vi "RelaySafetyTest.vi"(0 "Relay Task":refnum<k21>, 5 "task error in":errorcluster, 9 "NI VISA":refnum<visa-resource-name>, 11 "NHR error in":errorcluster caption="error in (no error)") -> (6 "error out":errorcluster, 8 "Safe to connect":bool, 10 "NHR Visa out":refnum<visa-resource-name>, 15 "NHR error out":errorcluster)   [LabVIEW 2020]
uses:
  <vilib>/DAQmx/write.llb/DAQmx Write (Digital 1D Bool NChan 1Samp 1Line).vi
  <vilib>/DAQmx/miscellaneous.llb/DAQmx Fill In Error Info.vi
  <instrlib>/NH Research Regenerative Test Series/Public/Data/Read (Ave Voltage).vi
  <instrlib>/NH Research Regenerative Test Series/NH Research Regenerative Test Series.lvlib
panel:
  out "Ave Voltage (V) 3":dbl
  out "Ave Voltage (V) 2":dbl
  out "Ave Voltage (V) 1":dbl
  in  "Logical Instrument Number":u32=1
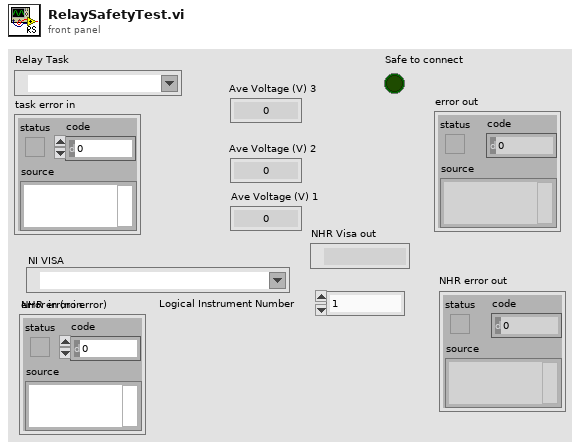
[diagram p1: front panel]
types:
  T1 = cluster{"Min Voltage (V)":dbl, "Min Voltage Time (s)":dbl, "Max Voltage (V)":dbl, "Max Voltage Time (s)":dbl, "Max Sink Current (A)":dbl, "Max Sink Current Time (s)":dbl, "Max Source Current (A)":dbl, "Max Source Current Time (s)":dbl, "Max Sink Power (W)":dbl, "Max Sink Power Time (s)":dbl, "Max Source Power (W)":dbl, "Max Source Power Time (s)":dbl}
  T2 = cluster{bool, bool, bool, bool, bool, bool, bool}
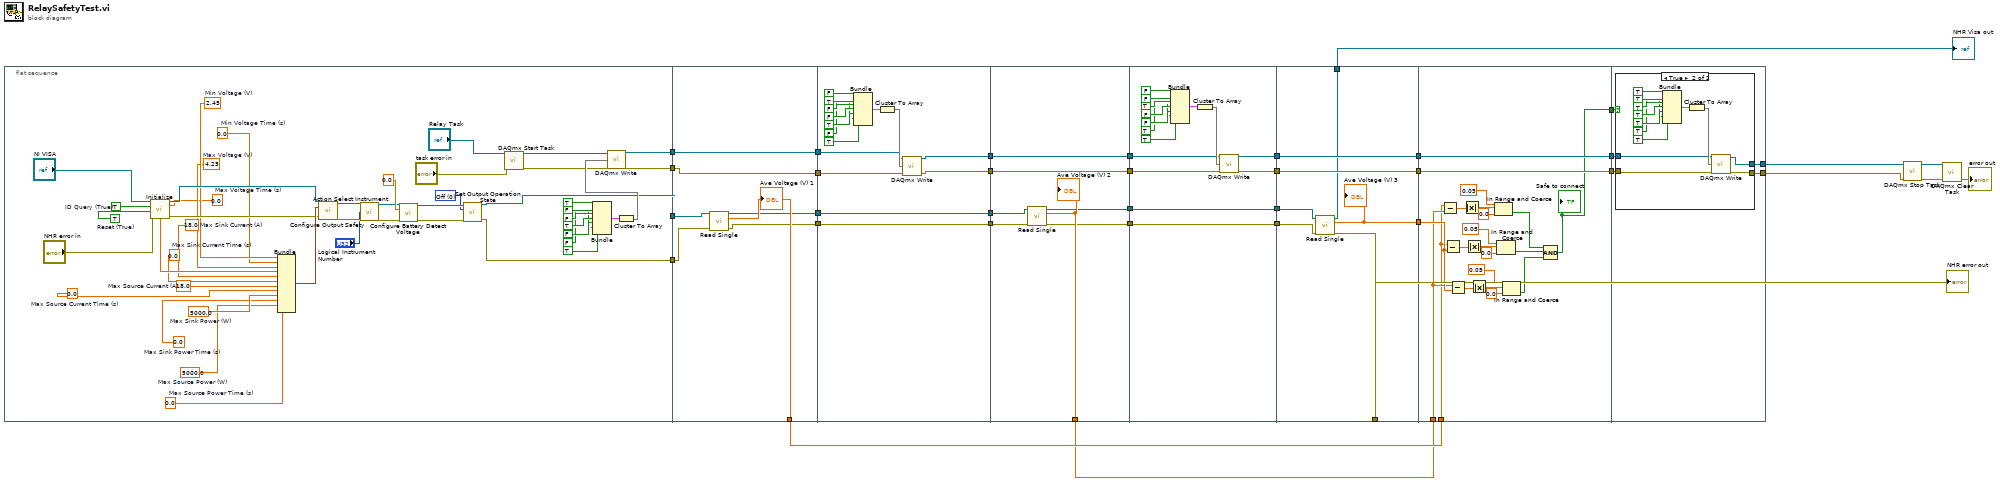
[diagram p0: block diagram]
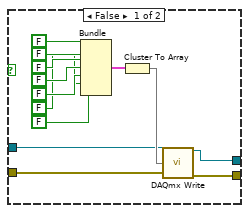
[diagram p2: hidden frame]
diagram:
  n1 = flat-sequence {
    tunnel: [w40] -> w35
    tunnel: [w39] -> w34
    tunnel: [w38] -> w33
    tunnel: [w37] -> w32
    tunnel: w35 -> [w82]
    tunnel: w34 -> [w81]
    tunnel: w33 -> [w87]
    tunnel: w32 -> [w86]
    tunnel: [w85] -> w31
    tunnel: [w84] -> w24
    tunnel: [w83] -> w22
    tunnel: [w82] -> w4
    tunnel: [w81] -> w3
    tunnel: [w93] -> w25
    tunnel: w24 -> [w93]
    tunnel: [w92] -> w23
    tunnel: w22 -> [w92]
    tunnel: [w91] -> w20
    tunnel: [w90] -> w18
    tunnel: w4 -> [w89]
    tunnel: w3 -> [w88]
    tunnel: [w109] -> w30
    tunnel: w25 -> [w108]
    tunnel: w23 -> [w107]
    tunnel: [w106] -> w21
    tunnel: w20 -> [w106]
    tunnel: [w105] -> w19
    tunnel: w18 -> [w105]
    tunnel: [w104] -> w16
    tunnel: [w103] -> w14
    tunnel: w21 -> [w115]
    tunnel: w19 -> [w114]
    tunnel: [w113] -> w17
    tunnel: w16 -> [w113]
    tunnel: [w112] -> w15
    tunnel: w14 -> [w112]
    tunnel: [w111] -> w11
    tunnel: [w110] -> w8
    tunnel: [w131] -> w29
    tunnel: w17 -> [w130]
    tunnel: w15 -> [w129]
    tunnel: [w128] -> w12
    tunnel: w11 -> [w128]
    tunnel: [w127] -> w9
    tunnel: w8 -> [w127]
    tunnel: [w126] -> w2
    tunnel: [w125] -> w1
    tunnel: w31 -> [w135]
    tunnel: w30 -> [w136]
    tunnel: w29 -> [w137]
    tunnel: [w134] -> w13
    tunnel: w12 -> [w134]
    tunnel: [w133] -> w10
    tunnel: w9 -> [w133]
    tunnel: [w132] -> w5
    tunnel: w13 -> [w157]
    tunnel: w10 -> [w156]
    tunnel: [w155] -> w7
    tunnel: [w154] -> w6
    tunnel: w5 -> [w153]
    frame #0 {
      w52 = 0 items=["Off", "Standby", "Charge", "Discharge", "Battery"] ("Mode (0: Off)")
      w71 = TRUE  # ID Query (True)
      w70 = TRUE  # Reset (True)
      w59 = 5000.0  # Max Source Power (W)
      w60 = 0.0  # Max Sink Power Time (s)
      w61 = 5000.0  # Max Sink Power (W)
      w62 = 0.0  # Max Source Current Time (s)
      w63 = 18.0  # Max Source Current (A)
      w65 = 18.0  # Max Sink Current (A)
      w64 = 0.0  # Max Sink Current Time (s)
      w66 = 0.0  # Max Voltage Time (s)
      w67 = 4.25  # Max Voltage (V)
      w69 = 2.45  # Min Voltage (V)
      w58 = 0.0  # Max Source Power Time (s)
      w68 = 0.0  # Min Voltage Time (s)
      n2 = call <instrlib>:"Initialize.vi"("VISA resource name"="NI VISA", "ID Query (True)"=w71, "Reset (True)"=w70, "error in (no error)"="NHR error in") -> ("VISA resource name out"=w73:refnum<visa-resource-name>, "error out"=w74:errorcluster)  [unwired: 10 in]
      n3 = Bundle("Min Voltage (V)"=w69, "Min Voltage Time (s)"=w68, "Max Voltage (V)"=w67, "Max Voltage Time (s)"=w66, "Max Sink Current (A)"=w65, "Max Sink Current Time (s)"=w64, "Max Source Current (A)"=w63, "Max Source Current Time (s)"=w62, "Max Sink Power (W)"=w61, "Max Sink Power Time (s)"=w60, "Max Source Power (W)"=w59, "Max Source Power Time (s)"=w58) -> (w75:T1)  [unwired: 1 in]
      n4 = call <instrlib>:"Configure Output Safety.vi"("VISA resource name"=w73, "Output Safety"=w75, "error in (no error)"=w74) -> ("VISA resource name out"=w77:refnum<visa-resource-name>, "error out"=w78:errorcluster)  [unwired: 11 in]
      n5 = call <instrlib>:"Action Select Instrument.vi"("VISA resource name"=w77, "Logical Instrument Number"="Logical Instrument Number", "error in (no error)"=w78) -> ("VISA resource name out"=w56:refnum<visa-resource-name>, "error out"=w55:errorcluster)  [unwired: 11 in]
      n6 = call <instrlib>:"Configure Battery Detect Voltage.vi"("VISA resource name"=w56, "Battery Detect Voltage (0V)"=0.0, "error in (no error)"=w55) -> ("VISA resource name out"=w54:refnum<visa-resource-name>, "error out"=w53:errorcluster)  [unwired: 11 in]
      n7 = call <vilib>:"Set Output Operation State.vi"("VISA resource name"=w54, "Mode (0: Off)"=w52, "error in (no error)"=w53) -> ("VISA resource name out"=w38:refnum<visa-resource-name>, "error out"=w37:errorcluster)  [unwired: 11 in]
      n8 = call <vilib>:"DAQmx Start Task.vi"("task/channels in"="Relay Task", "error in"="task error in") -> ("task out"=w42:refnum<k21>, "error out"=w41:errorcluster)  [unwired: 12 in]
      n9 = Bundle(TRUE, FALSE, FALSE, TRUE, FALSE, FALSE, TRUE) -> (w51:T2)  [unwired: 1 in]
      n10 = Cluster To Array(cluster=w51) -> (array=w43:bool[])
      n11 = call-poly <vilib>:"DAQmx Write.vi"("task/channels in"=w42, "data"=w43, "error in"=w41) -> ("task out"=w40:refnum<k21>, "error out"=w39:errorcluster)  [unwired: 10 in, 1 out]
    }
    frame #1 {
      n12 = call-poly <instrlib>:"Read Single.vi"("VISA resource name"=w87, "error in (no error)"=w86) -> ("VISA resource name out"=w84:refnum<visa-resource-name>, "Ave Voltage (V)"=w85:dbl, "error out"=w83:errorcluster)  [unwired: 11 in]
      "Ave Voltage (V) 1" <- w85
    }
    frame #2 {
      n13 = Bundle(FALSE, TRUE, FALSE, FALSE, TRUE, FALSE, TRUE) -> (w102:T2)  [unwired: 1 in]
      n14 = Cluster To Array(cluster=w102) -> (array=w94:bool[])
      n15 = call-poly <vilib>:"DAQmx Write.vi"("task/channels in"=w89, "data"=w94, "error in"=w88) -> ("task out"=w91:refnum<k21>, "error out"=w90:errorcluster)  [unwired: 10 in, 1 out]
    }
    frame #3 {
      n16 = call-poly <instrlib>:"Read Single.vi"("VISA resource name"=w108, "error in (no error)"=w107) -> ("VISA resource name out"=w104:refnum<visa-resource-name>, "Ave Voltage (V)"=w109:dbl, "error out"=w103:errorcluster)  [unwired: 11 in]
      "Ave Voltage (V) 2" <- w109
    }
    frame #4 {
      n17 = Bundle(FALSE, FALSE, TRUE, FALSE, FALSE, TRUE, TRUE) -> (w124:T2)  [unwired: 1 in]
      n18 = Cluster To Array(cluster=w124) -> (array=w116:bool[])
      n19 = call-poly <vilib>:"DAQmx Write.vi"("task/channels in"=w115, "data"=w116, "error in"=w114) -> ("task out"=w111:refnum<k21>, "error out"=w110:errorcluster)  [unwired: 10 in, 1 out]
    }
    frame #5 {
      n20 = call-poly <instrlib>:"Read Single.vi"("VISA resource name"=w130, "error in (no error)"=w129) -> ("VISA resource name out"=w126:refnum<visa-resource-name>, "Ave Voltage (V)"=w131:dbl, "error out"=w125:errorcluster)  [unwired: 11 in]
      "Ave Voltage (V) 3" <- w131
    }
    frame #6 {
      n21 = Subtract(x=w135, y=w136) -> (x-y=w152:dbl)
      n22 = Subtract(x=w135, y=w137) -> (x-y=w148:dbl)
      n23 = Subtract(x=w136, y=w137) -> (x-y=w144:dbl)
      n24 = Absolute Value(x=w152) -> (abs(x)=w149:dbl)
      n25 = Absolute Value(x=w148) -> (abs(x)=w145:dbl)
      n26 = Absolute Value(x=w144) -> (abs(x)=w141:dbl)
      n27 = In Range and Coerce(upper limit=0.05, x=w149, lower limit=0.0) -> (In Range?=w140:bool)  [unwired: 1 out]
      n28 = In Range and Coerce(upper limit=0.05, x=w145, lower limit=0.0) -> (In Range?=w139:bool)  [unwired: 1 out]
      n29 = In Range and Coerce(upper limit=0.05, x=w141, lower limit=0.0) -> (In Range?=w138:bool)  [unwired: 1 out]
      n30 = Compound Arithmetic op=AND(w140, w139, w138) -> (w132:bool)
      "Safe to connect" <- w132
    }
    frame #7 {
      n31 = case shown="True" w153 {
        tunnel: w157 -> [w161 w174]
        tunnel: w156 -> [w160 w173]
        tunnel: [w159 w172] -> w155
        tunnel: [w158 w171] -> w154
        frame False {
          n32 = Bundle(FALSE, FALSE, FALSE, FALSE, FALSE, FALSE, FALSE) -> (w170:T2)  [unwired: 1 in]
          n33 = Cluster To Array(cluster=w170) -> (array=w162:bool[])
          n34 = call-poly <vilib>:"DAQmx Write.vi"("task/channels in"=w161, "data"=w162, "error in"=w160) -> ("task out"=w159:refnum<k21>, "error out"=w158:errorcluster)  [unwired: 10 in, 1 out]
        }
        frame True {
          n35 = Bundle(TRUE, TRUE, TRUE, TRUE, TRUE, TRUE, TRUE) -> (w183:T2)  [unwired: 1 in]
          n36 = Cluster To Array(cluster=w183) -> (array=w175:bool[])
          n37 = call-poly <vilib>:"DAQmx Write.vi"("task/channels in"=w174, "data"=w175, "error in"=w173) -> ("task out"=w172:refnum<k21>, "error out"=w171:errorcluster)  [unwired: 10 in, 1 out]
        }
      }
    }
  }
  n38 = call <vilib>:"DAQmx Stop Task.vi"("task/channels in"=w7, "error in"=w6) -> ("task out"=w28:refnum<k21>, "error out"=w27:errorcluster)  [unwired: 12 in]
  n39 = call <vilib>:"DAQmx Clear Task.vi"("task in"=w28, "error in"=w27) -> ("error out"=→"error out":errorcluster)  [unwired: 13 in]
  "NHR Visa out" <- w2
  "NHR error out" <- w1
